vi "Write Power.vi"(8 "error in":errorcluster, 10 "Power":sgl, 11 "Change Meerstetter Power in":refnum<class "Change Meerstetter Power.lvclass">) -> (0 "error out":errorcluster, 3 "Change Meerstetter Power out":refnum<class "Change Meerstetter Power.lvclass">)   [LabVIEW 2014, in "Meerstetter Lib.lvlib" / "Change Meerstetter Power.lvclass"]
uses:
  Change Meerstetter Power.lvclass
  Change Meerstetter Power.lvclass/Change Meerstetter Power.ctl
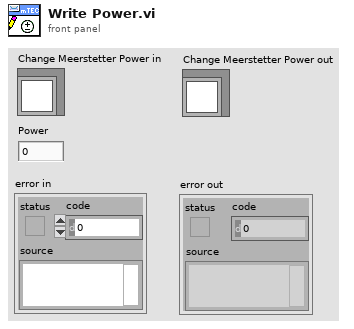
[diagram p1: front panel]
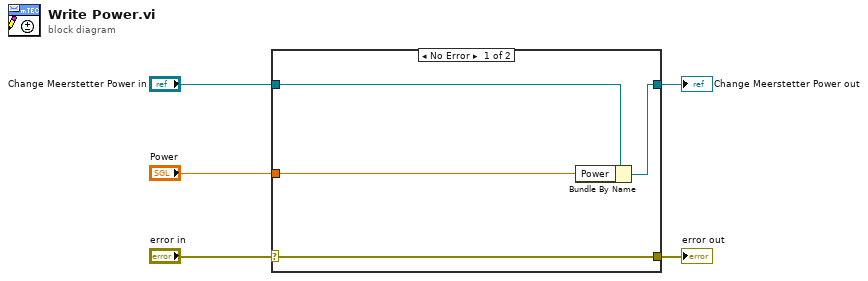
[diagram p0: block diagram]
diagram:
  n1 = case shown="No Error" "error in" {
    selector: "error in" -> [w9 w10]
    tunnel: [w9 w10] -> w4
    tunnel: [w7 w11] -> w2
    tunnel: "Change Meerstetter Power in" -> [w8 w11]
    tunnel: "Power" -> [w6 _]
    frame No Error {
      n2 = Bundle By Name(cluster=w8, "Power"=w6) -> (w7:refnum<class "Change Meerstetter Power.lvclass">)
    }
    frame Error {
    }
  }
  "error out" <- w4
  "Change Meerstetter Power out" <- w2
